vi "Generate Track ROI.vi"(8 "error in (no error)":errorcluster, 9 "ROI Width":dbl=50.0, 10 "Tip 2":T2={"Point"={"X"=0.0, "Y"=0.0}, "Angle"=0.0, "Frame Number"=0, "ROI Descriptor"={"Global Rectangle"=[], "Contours"=[]}, "Curvature"=0.0, "Label"="Non-tip"} {"ROI Descriptor"."Contours"."Type" items=["No Selection", "Point", "Line", "Rectangle", "Oval", "Polygon", "Freehand Region", "Annulus", "Unused2", "Unused3", "Broken Line", "Freehand Line", "Rotated Rectangle"]; "Point"."Y" format="%.2f"; "Point"."X" format="%.2f"}, 11 "Tip 1":T2={"Point"={"X"=0.0, "Y"=0.0}, "Angle"=0.0, "Frame Number"=0, "ROI Descriptor"={"Global Rectangle"=[], "Contours"=[]}, "Curvature"=0.0, "Label"="Non-tip"} {"ROI Descriptor"."Contours"."Type" items=["No Selection", "Point", "Line", "Rectangle", "Oval", "Polygon", "Freehand Region", "Annulus", "Unused2", "Unused3", "Broken Line", "Freehand Line", "Rotated Rectangle"]; "Point"."Y" format="%.2f"; "Point"."X" format="%.2f"}) -> (0 "error out":errorcluster, 3 "Track ROI":T1 {"Contours"."Type" items=["No Selection", "Point", "Line", "Rectangle", "Oval", "Polygon", "Freehand Region", "Annulus", "Unused2", "Unused3", "Broken Line", "Freehand Line", "Rotated Rectangle"]})   [LabVIEW 2013]
uses:
  Controls/Tip.ctl
  <vilib>/vision/NI_Vision_Development_Module.lvlib
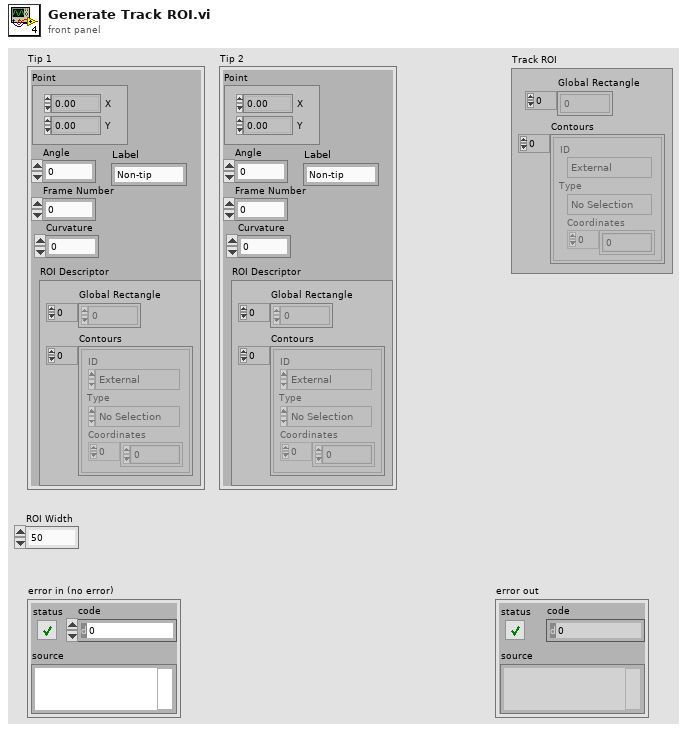
[diagram p1: front panel]
types:
  T1 = typedef "ROI Descriptor" = cluster{"Global Rectangle":i32[], "Contours":cluster{"ID":enum32{"External", "Internal"}, "Type":u32, "Coordinates":i32[]}[]}
  T2 = typedef "Tip.ctl" = cluster{"Point":T3, "Angle":dbl, "Frame Number":i32, "ROI Descriptor":T1, "Curvature":dbl, "Label":string}
  T3 = typedef "IMAQ Point" = cluster{"X":sgl, "Y":sgl}
  T4 = typedef "IMAQ Rectangle" = cluster{"Left":i32, "Top":i32, "Right":i32, "Bottom":i32, "Rotation":dbl}
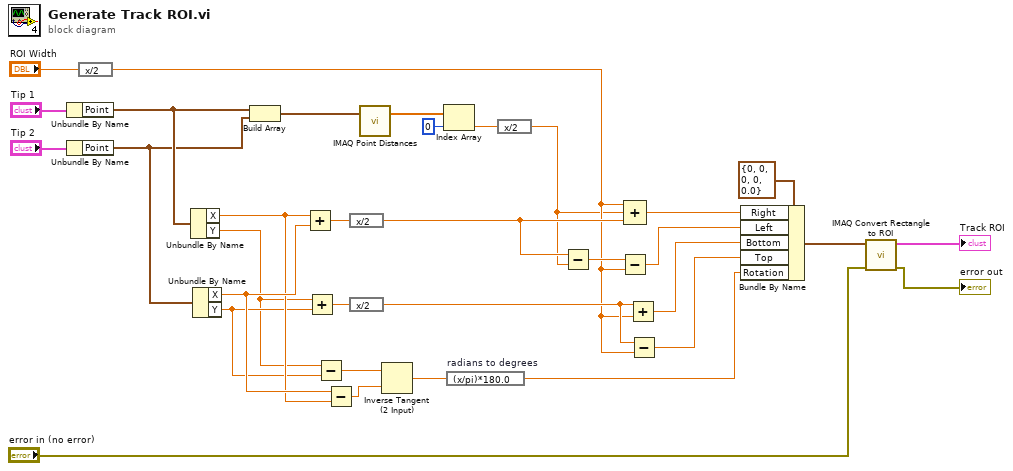
[diagram p0: block diagram]
diagram:
  n1 = Unbundle By Name("Tip 1") -> ("Point"=w26:T3)
  n2 = Unbundle By Name("Tip 2") -> ("Point"=w25:T3)
  n3 = expression code="x/2"("ROI Width") -> (w17:dbl)
  n4 = Unbundle By Name(w26) -> ("X"=w11:sgl, "Y"=w5:sgl)
  n5 = Unbundle By Name(w25) -> ("X"=w12:sgl, "Y"=w6:sgl)
  n6 = Build Array(w26, w25) -> (w31:T3[])
  n7 = Add(x=w11, y=w12) -> (x+y=w28:sgl)
  n8 = Add(x=w5, y=w6) -> (x+y=w27:sgl)
  n9 = Subtract(x=w5, y=w6) -> (x-y=w10:sgl)
  n10 = Subtract(x=w12, y=w11) -> (x-y=w9:sgl)
  n11 = expression code="x/2"(w28) -> (w23:sgl)
  n12 = expression code="x/2"(w27) -> (w18:sgl)
  n13 = call "IMAQ Point Distances"("Points"=w31) -> ("Distances"=w30:sgl[])  [unwired: 4 in, 1 out]
  n14 = Inverse Tangent (2 Input)(1:w9, 2:w10) -> (0:w4:sgl)
  n15 = Index Array(array=w30, index=0) -> (element=w2:sgl)
  n16 = expression code="(x/pi)*180.0" "radians to degrees"(w4) -> (w3:sgl)
  n17 = expression code="x/2"(w2) -> (w1:sgl)
  n18 = Subtract(x=w23, y=w1) -> (x-y=w22:sgl)
  n19 = Subtract(x=w22, y=w17) -> (x-y=w19:dbl)
  n20 = Compound Arithmetic op=ADD(w17, w1, w23) -> (w20:dbl)
  n21 = Add(x=w18, y=w17) -> (x+y=w16:dbl)
  n22 = Subtract(x=w18, y=w17) -> (x-y=w15:dbl)
  n23 = Bundle By Name(cluster=T4 {"Left"=0, "Top"=0, "Right"=0, "Bottom"=0, "Rotation"=0.0} ("Rectangle"), "Right"=w20, "Left"=w19, "Bottom"=w16, "Top"=w15, "Rotation"=w3) -> (w14:T4)
  n24 = call "IMAQ Convert Rectangle to ROI"("error in (no error)"="error in (no error)", "Rectangle"=w14) -> ("error out"=→"error out":errorcluster, "ROI Descriptor"=→"Track ROI":T1)  [unwired: 7 in]
